vi "控制曲线是否可见（数据流）.vi"() -> ()   [LabVIEW 2012]
uses:
  <vilib>/measure/NI_MABase.lvlib
panel:
  out "波形图":waveform(dbl)[](graph)
  in  "Active":bool[](array[boolean])
  in  "stop":bool
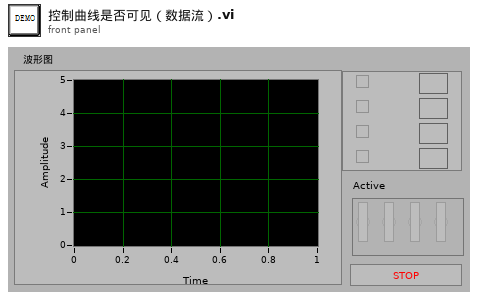
[diagram p1: front panel]
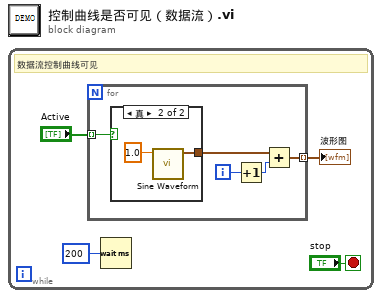
[diagram p0: block diagram]
diagram:
  n1 = while "While循环" {
    stop <- "stop" stop-if-true
    # "数据流控制曲线可见"
    n2 = for {
      tunnel: "Active" -> [w9] mode=indexing
      tunnel: [w5] -> w1 mode=indexing
      i -> [w8]
      n3 = case shown="真" w9 {
        tunnel: [_ w11] -> w6
        frame False {
        }
        frame True {
          n4 = call <vilib>:"Sine Waveform.vi"("frequency"=1.0) -> ("signal out"=w11:waveform(dbl))  [unwired: 9 in, 1 out]
        }
      }
      n5 = Increment(x=w8) -> (x+1=w7:i32)
      n6 = Add(x=w6, y=w7) -> (x+y=w5:waveform(dbl))
    }
    "波形图" <- w1
    n7 = Wait (ms)(milliseconds to wait=u32 200 ("等待时间（毫秒）")) -> ()  [unwired: 1 out]
  }
